vi "Start AWG.vi"(8 "error in (no error)":errorcluster, 11 "AWG":T1={"AWG type"=enum."Agilent 331xxA to 332xxA", "FGEN Resource Name"="", "Source (Onboard Clock)"="OnboardClock", "FGEN Channel"="0", "awg lib session"={"type"=enum."Agilent 331xxA to 332xxA", "VISA"="", "enable 10MHz ref"=FALSE, "cmi ckd2"={"VISA"="", "clock source"=enum."Auto", "manual ref clk"=FALSE, "ref clock [Hz]"=0.0, "div mode"=enum."Set divisor directly"}, "cmi sync v3"={"VISA"="", "baud rate [bd/s]"=115200, "source"=enum."Auto", "hv range"=enum."1kV", "fsrc is fixed"=FALSE, "fsrc [Hz]"=10000000.0, "freq integ [s]"=1.0, "freq filter"=5, "trig level"=enum."TTL 5V", "chn1 mode"=enum."Source divider", "chn1 level"=enum."Positive 5V", "chn2 mode"=enum."Source divider", "chn2 level"=enum."Positive 5V", "chn2 div"=1, "chn3 mode"=enum."Chn 1 Active", "chn3 level"=enum."Positive 5V", "chn1 div entry"=enum."Calculate nearest divisor from measured fx", "chn1 dev limit [%]"=1.0, "chn1 check dev"=FALSE}, "trigger"={"source"=enum."Immediate", "level [V]"=0.0, "coupling"=enum."DC", "slope"=enum."POS"}, "HMF2500 cfg"={"Baud Rate"=9600, "Parity"=0, "Data Bits"=8, "Flow Control"=4}}} {"awg lib session"."HMF2500 cfg"."Flow Control" items=["None", "XON/XOFF", "RTS/CTS", "XON/XOFF & RTS/CTS", "DTR/DSR", "XON/XOFF & DTR/DSR"]; "awg lib session"."HMF2500 cfg"."Data Bits" items=["7"=7, "8"=8]; "awg lib session"."HMF2500 cfg"."Parity" items=["None", "Odd", "Even", "Mark", "Space"]; "awg lib session"."HMF2500 cfg"."Baud Rate" items=["300"=300, "600"=600, "1200"=1200, "2400"=2400, "4800"=4800, "9600"=9600, "19200"=19200]; "awg lib session"."cmi sync v3"."chn2 div" min=1 max=100000000 step=1; "awg lib session"."cmi sync v3"."fsrc [Hz]" format="%_8p"}) -> (0 "error out":errorcluster, 3 "AWG out":T1={"AWG type"=enum."Agilent 331xxA to 332xxA", "FGEN Resource Name"="", "Source (Onboard Clock)"="OnboardClock", "FGEN Channel"="0", "awg lib session"={"type"=enum."Agilent 331xxA to 332xxA", "VISA"="", "enable 10MHz ref"=FALSE, "cmi ckd2"={"VISA"="", "clock source"=enum."Auto", "manual ref clk"=FALSE, "ref clock [Hz]"=0.0, "div mode"=enum."Set divisor directly"}, "cmi sync v3"={"VISA"="", "baud rate [bd/s]"=115200, "source"=enum."Auto", "hv range"=enum."1kV", "fsrc is fixed"=FALSE, "fsrc [Hz]"=10000000.0, "freq integ [s]"=1.0, "freq filter"=5, "trig level"=enum."TTL 5V", "chn1 mode"=enum."Source divider", "chn1 level"=enum."Positive 5V", "chn2 mode"=enum."Source divider", "chn2 level"=enum."Positive 5V", "chn2 div"=1, "chn3 mode"=enum."Chn 1 Active", "chn3 level"=enum."Positive 5V", "chn1 div entry"=enum."Calculate nearest divisor from measured fx", "chn1 dev limit [%]"=1.0, "chn1 check dev"=FALSE}, "trigger"={"source"=enum."Immediate", "level [V]"=0.0, "coupling"=enum."DC", "slope"=enum."POS"}, "HMF2500 cfg"={"Baud Rate"=9600, "Parity"=0, "Data Bits"=8, "Flow Control"=4}}} {"awg lib session"."HMF2500 cfg"."Flow Control" items=["None", "XON/XOFF", "RTS/CTS", "XON/XOFF & RTS/CTS", "DTR/DSR", "XON/XOFF & DTR/DSR"]; "awg lib session"."HMF2500 cfg"."Data Bits" items=["7"=7, "8"=8]; "awg lib session"."HMF2500 cfg"."Parity" items=["None", "Odd", "Even", "Mark", "Space"]; "awg lib session"."HMF2500 cfg"."Baud Rate" items=["300"=300, "600"=600, "1200"=1200, "2400"=2400, "4800"=4800, "9600"=9600, "19200"=19200]; "awg lib session"."cmi sync v3"."chn2 div" min=1 max=100000000 step=1; "awg lib session"."cmi sync v3"."fsrc [Hz]" format="%_8p"})   [LabVIEW 2020]
uses:
  Type definitions/AWG.ctl
  Type definitions/AWG type.ctl
  <instrlib>/niFgen/niFgen.llb/niFgen_ctl Sample Clock Source Values (Ring).ctl
  external libraries/AWG/AWG Session.ctl
  external libraries/AWG/AWG Type.ctl
  external libraries/AWG/CMI Clock Divider v2/CMI ckd2 Session.ctl
  external libraries/AWG/CMI Clock Divider v2/CMI ckd2 Source Mode.ctl
  external libraries/AWG/CMI Clock Divider v2/CMI ckd2 Divisor Mode.ctl
  external libraries/AWG/CMI Sync V3/CMI Sync V3 session.ctl
  external libraries/AWG/CMI Sync V3/Configure/CMI Sync V3 Reference Clock Source.ctl
  external libraries/AWG/CMI Sync V3/Configure/CMI Sync V3 HV input Range.ctl
  external libraries/AWG/CMI Sync V3/Configure/CMI Sync V3 Trigger Input Level.ctl
  external libraries/AWG/CMI Sync V3/Configure/CMI Sync V3 Channel 1 Mode.ctl
  external libraries/AWG/CMI Sync V3/Configure/CMI Sync V3 Channel Output Levels.ctl
  external libraries/AWG/CMI Sync V3/Configure/CMI Sync V3 Channel 2 Mode.ctl
  external libraries/AWG/CMI Sync V3/Configure/CMI Sync V3 Channel 3 Mode.ctl
  external libraries/AWG/CMI Sync V3/Configure/CMI Sync V3 Channel 1 Divisor Entry Mode.ctl
  external libraries/AWG/RaS HMF2500/HMF2500 Config.ctl
  external libraries/AWG/AWG.lvlib
  external libraries/AWG/CMI Sync V3/CMI Sync Unit V3.lvlib
  external libraries/externals needed for AWG/ADC Trig Mode Source.ctl
  external libraries/externals needed for AWG/ADC Trig Coupling.ctl
  external libraries/externals needed for AWG/ADC Trig Slope.ctl
  external libraries/externals needed for AWG/ADC Trig Config.ctl
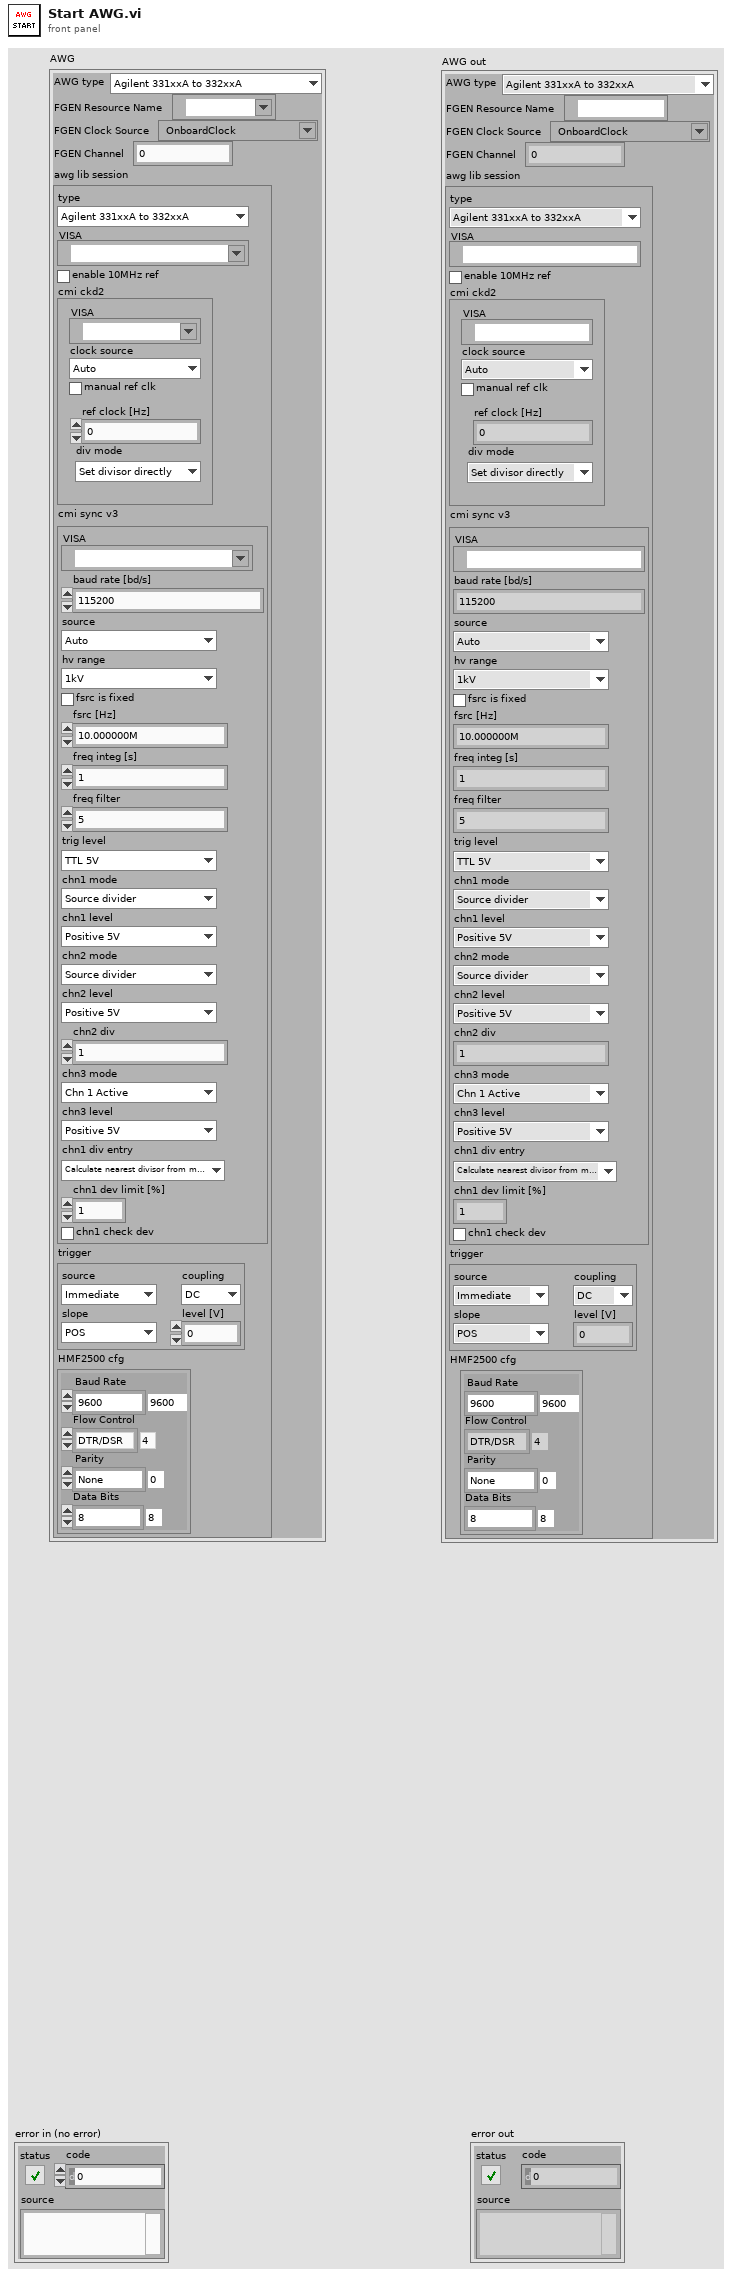
[diagram p1: front panel]
types:
  T1 = typedef "AWG.ctl" = cluster{"AWG type":T2, "FGEN Resource Name":refnum<k15>, "Source (Onboard Clock)":T3, "FGEN Channel":string, "awg lib session":T4}
  T2 = typedef "AWG type.ctl" = enum16{"Agilent 331xxA to 332xxA", "Agilent 335xxA to 336xxA", "Tektronix AFG3101C", "R&S HMF25xx", "CMI Clock Divider v2", "CMI Sync Unit V3", "FGEN NI 5413", "Supracon PJVS Generator", "dummy"}
  T3 = typedef "niFgen_ctl Sample Clock Source Values (Ring).ctl" = string
  T4 = typedef "AWG.lvlib/AWG Session.ctl" = cluster{"type":T5, "VISA":refnum<visa-resource-name>, "enable 10MHz ref":bool, "cmi ckd2":T6, "cmi sync v3":T9, "trigger":T18, "HMF2500 cfg":T22}
  T5 = typedef "AWG.lvlib/AWG Type.ctl" = enum16{"Agilent 331xxA to 332xxA", "Agilent 335xxA to 336xxA", "Tektronix AFG3101C", "R&S HMF25xx", "CMI Clock Divider v2", "CMI Sync Unit V3", "dummy"}
  T6 = typedef "AWG.lvlib/CMI ckd2 Session.ctl" = cluster{"VISA":refnum<visa-resource-name>, "clock source":T7, "manual ref clk":bool, "ref clock [Hz]":dbl, "div mode":T8}
  T7 = typedef "AWG.lvlib/CMI ckd2 Source Mode.ctl" = enum16{"Auto", "LF clock", "HF clock", "Internal"}
  T8 = typedef "AWG.lvlib/CMI ckd2 Divisor Mode.ctl" = enum16{"Set divisor directly", "Set divisor by frequency"}
  T9 = typedef "AWG.lvlib/CMI Sync Unit V3.lvlib/CMI Sync V3 session.ctl" = cluster{"VISA":refnum<visa-resource-name>, "baud rate [bd/s]":i32, "source":T10, "hv range":T11, "fsrc is fixed":bool, "fsrc [Hz]":dbl, "freq integ [s]":dbl, "freq filter":i32, "trig level":T12, "chn1 mode":T13, "chn1 level":T14, "chn2 mode":T15, "chn2 level":T14, "chn2 div":i32, "chn3 mode":T16, "chn3 level":T14, "chn1 div entry":T17, "chn1 dev limit [%]":dbl, "chn1 check dev":bool}
  T10 = typedef "AWG.lvlib/CMI Sync Unit V3.lvlib/CMI Sync V3 Reference Clock Source.ctl" = enum16{"Auto", "Internal", "Logic", "Sine", "HV"}
  T11 = typedef "AWG.lvlib/CMI Sync Unit V3.lvlib/CMI Sync V3 HV input Range.ctl" = enum16{"10V", "60V", "250V", "1kV"}
  T12 = typedef "AWG.lvlib/CMI Sync Unit V3.lvlib/CMI Sync V3 Trigger Input Level.ctl" = enum16{"LVCMOS 3V3", "TTL 5V"}
  T13 = typedef "AWG.lvlib/CMI Sync Unit V3.lvlib/CMI Sync V3 Channel 1 Mode.ctl" = enum16{"Source divider", "DDS absolute", "DDS ratio", "DDS ratio M/N"}
  T14 = typedef "AWG.lvlib/CMI Sync Unit V3.lvlib/CMI Sync V3 Channel Output Levels.ctl" = enum16{"Positive 3V3", "Negative 3V3", "Positive 5V", "Negative 5V"}
  T15 = typedef "AWG.lvlib/CMI Sync Unit V3.lvlib/CMI Sync V3 Channel 2 Mode.ctl" = enum16{"Source divider", "Chn 1 divide"}
  T16 = typedef "AWG.lvlib/CMI Sync Unit V3.lvlib/CMI Sync V3 Channel 3 Mode.ctl" = enum16{"Chn 1 Active", "Chn 2 Active", "Chn 1 Trigger", "Chn 2 Trigger", "Gate", "PPS", "10MHz"}
  T17 = typedef "AWG.lvlib/CMI Sync Unit V3.lvlib/CMI Sync V3 Channel 1 Divisor Entry Mode.ctl" = enum16{"Set divisor directly", "Calculate nearest divisor from measured fx"}
  T18 = typedef "ADC Trig Config.ctl" = cluster{"source":T19, "level [V]":dbl, "coupling":T20, "slope":T21}
  T19 = typedef "ADC Trig Mode Source.ctl" = enum16{"Immediate", "External", "Level"}
  T20 = typedef "ADC Trig Coupling.ctl" = enum16{"DC", "AC"}
  T21 = typedef "ADC Trig Slope.ctl" = enum16{"POS", "NEG"}
  T22 = typedef "AWG.lvlib/HMF2500 Config.ctl" = cluster{"Baud Rate":u32, "Parity":u16, "Data Bits":u16, "Flow Control":u16}
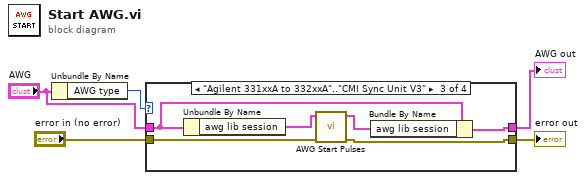
[diagram p0: block diagram]
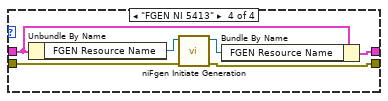
[diagram p4: hidden frame]
diagram:
  n1 = Unbundle By Name("AWG") -> ("AWG type"=w3:T2)
  n2 = case shown="\"Agilent 331xxA to 332xxA\"..\"CMI Sync Unit V3\"" w3 {
    tunnel: "error in (no error)" -> [w7 w9 w15 w17]
    tunnel: [w7 w9 w14 w16] -> w4
    tunnel: "AWG" -> [w6 w8 w10 w21]
    tunnel: [w6 w8 w11 w20] -> w1
    frame "Supracon PJVS Generator" {
      # "#2DO"
    }
    frame "dummy" {
    }
    frame "Agilent 331xxA to 332xxA".."CMI Sync Unit V3" {
      n3 = Unbundle By Name(w10) -> ("awg lib session"=w12:T4)
      n4 = call "AWG Start Pulses.vi"("error in (no error)"=w15, "awg session in"=w12) -> ("error out"=w14:errorcluster, "awg session out"=w13:T4)  [unwired: 8 in]
      n5 = Bundle By Name(cluster=w10, "awg lib session"=w13) -> (w11:T1)
    }
    frame "FGEN NI 5413" {
      n6 = Unbundle By Name(w21) -> ("FGEN Resource Name"=w19:refnum<k15>)
      n7 = call <instrlib>:"niFgen Initiate Generation.vi"("error in (no error)"=w17, "Instrument Handle"=w19) -> ("error out"=w16:errorcluster, "Instrument Handle Out"=w18:refnum<k15>)  [unwired: 8 in]
      n8 = Bundle By Name(cluster=w21, "FGEN Resource Name"=w18) -> (w20:T1)
    }
  }
  "error out" <- w4
  "AWG out" <- w1
